vi "M9003Close.vi"(0 "HANDLE":i32) -> ()   [LabVIEW 2009]
uses:
  M9003api.dll
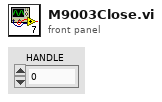
[diagram p1: front panel]
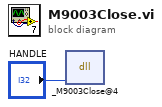
[diagram p0: block diagram]
diagram:
  n1 = dll-call lib="H:/Mover_2009/Sub_Vis/M9003Commands/M9003api.dll" fn="_M9003Close@4" label="M9003close"("Handle"="HANDLE") -> ()  [unwired: 4 in, 3 out]
